vi "test_RemoteDmmSession_CallInitializeMeasurementLinkSessionWithAttachBehavior_RemoteSessionAttached.vi"(8 "error in":errorcluster) -> (0 "error out":errorcluster, 2 "result":string, 3 "pass":bool)   [LabVIEW 2020, in "MeasurementServerTests.lvlib"]
uses:
  MeasurementServerTests.lvlib
  Runtime/MeasurementLink niDMM/Instrument/Session Factory.lvclass
  Runtime/MeasurementLink Instrument/ISession Factory/Initialize and Close Session Behavior.ctl
  Runtime/MeasurementLink Instrument/ISession Factory/ISession Factory.lvclass
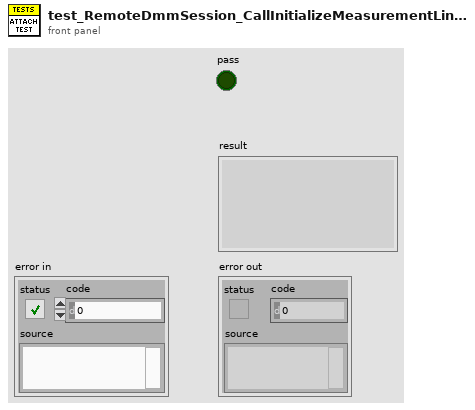
[diagram p1: front panel]
types:
  T1 = typedef "MeasurementLink Instrument.lvlib/ISession Factory.lvclass/Remote Connection Options.ctl" = cluster{"session name":string, "address":string, "port":u32}
  T2 = typedef "MeasurementLink Instrument.lvlib/ISession Factory.lvclass/Initialize and Close Session Behavior.ctl" = enum16{"Initialize and Close", "Attach and Detach", "Initialize and Detach", "Attach and Close"}
  T3 = typedef "MeasurementLink Instrument.lvlib/ISession Factory.lvclass/Session Initialization Parameters.ctl" = cluster{"resource name":string, "session name":string}
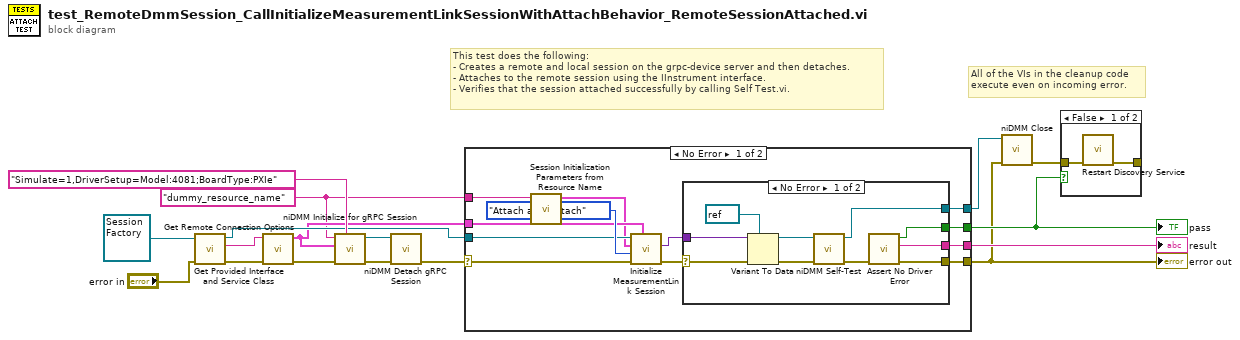
[diagram p0: block diagram]
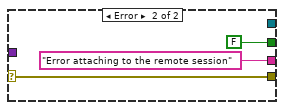
[diagram p2: hidden frame]
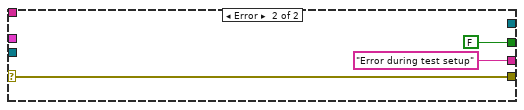
[diagram p3: hidden frame]
diagram:
  w2 = "dummy_resource_name" ("resource name")
  # "All of the VIs in the cleanup code\nexecute even on incoming error."
  # "This test does the following:\n- Creates a remote and local session on the grpc-device server and then detaches.\n- Attaches to the remote session using the IInstrument interface.\n- Verifies that the session attached successfully by calling Self Test.vi."
  n1 = call-dynamic "Get Provided Interface and Service Class.vi"("error in"="error in", "instrument in"=refnum<class "Session Factory.lvclass"> refnum ("MeasurementLink niDMM.lvlib:Instrument.lvclass")) -> ("error out"=w10:errorcluster, "provided interface"=w9:string, "instrument out"=w7:refnum<class "Session Factory.lvclass">)  [unwired: 6 in, 1 out]
  n2 = call "Get Remote Connection Options.vi"("error in"=w10, "provided interface"=w9) -> ("error out"=w11:errorcluster, "remote connection options"=w3:T1)  [unwired: 8 in]
  n3 = call <instrlib>:"niDMM Initialize for gRPC Session.vi"("Option String"="Simulate=1,DriverSetup=Model:4081;BoardType:PXIe" ("option string"), "error in (no error)"=w11, "gRPC Options"=w3, "Instrument Descriptor"=w2) -> ("error out"=w6:errorcluster, "instrument handle out"=w4:refnum<k15>)  [unwired: 6 in]
  n4 = call <instrlib>:"niDMM Detach gRPC Session.vi"("error in (no error)"=w6, "instrument handle"=w4) -> ("error out"=w5:errorcluster)  [unwired: 9 in]
  n5 = case shown="No Error" w5 {
    selector: w5 -> [w23 w43]
    tunnel: [w28 w43] -> w13
    tunnel: [w29 FALSE] -> w14
    tunnel: [w27 "Error during test setup" ("f")] -> w17
    tunnel: w7 -> [w22 _]
    tunnel: [w21 _] -> w16
    tunnel: w3 -> [w20 _]
    tunnel: w2 -> [w19 _]
    frame No Error {
      n6 = call "Session Initialization Parameters from Resource Name.vi"("resource name"=w19) -> ("session initialization parameters"=w18:T3)  [unwired: 10 in]
      n7 = call-dynamic "Initialize MeasurementLink Session.vi"("remote connection options"=w20, "error in"=w23, "initialize and close session behavior"=Initialize_and_Close_Session_Behavior."Attach and Detach", "session initialization parameters"=w18, "instrument in"=w22) -> ("error out"=w25:errorcluster, "session out"=w26:variant)  [unwired: 4 in, 1 out]
      n8 = case shown="No Error" w25 {
        selector: w25 -> [w38 w41]
        tunnel: [w34 FALSE] -> w29
        tunnel: [w32 w41] -> w28
        tunnel: [w33 "Error attaching to the remote session"] -> w27
        tunnel: w26 -> [w39 _]
        tunnel: [w36 _] -> w21
        frame No Error {
          n9 = Variant To Data(error in=w38, type=refnum<k15> refnum ("instrument handle"), Variant=w39) -> (data=w31:refnum<k15>, error out=w37:errorcluster)
          n10 = call <instrlib>:"niDMM Self-Test.vi"("error in (no error)"=w37, "instrument handle"=w31) -> ("error out"=w35:errorcluster, "instrument handle out"=w36:refnum<k15>)  [unwired: 6 in, 2 out]
          n11 = call "Assert No Driver Error.vi"("error in"=w35) -> ("error out"=w32:errorcluster, "result"=w33:string, "pass?"=w34:bool)  [unwired: 8 in]
        }
        frame Error {
        }
      }
    }
    frame Error {
    }
  }
  "error out" <- w13
  "pass" <- w14
  "result" <- w17
  n12 = call <instrlib>:"niDMM Close.vi"("error in (no error)"=w13, "instrument handle"=w16) -> ("error out"=w15:errorcluster)  [unwired: 9 in]
  n13 = case shown="False" w14 {
    tunnel: w15 -> [w47 _]
    tunnel: [w46 _] -> _
    frame False {
      n14 = call "Restart Discovery Service.vi"("error in"=w47) -> ("error out"=w46:errorcluster)  [unwired: 10 in]
    }
    frame True {
    }
  }
